vi "test_GetItemInformationFromProjects_SampleProject.vi"() -> (3 "Pass?":bool)   [LabVIEW 2019, in "Tests.SolutionBuilder.lvlib"]
uses:
  Tests.SolutionBuilder.lvlib
  SolutionBuilder/SolutionBuilder.lvclass
  SolutionBuilder/ProjectItem/ProjectItem.lvclass
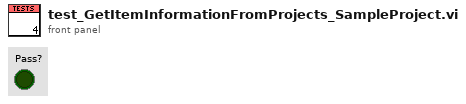
[diagram p1: front panel]
types:
  T1 = typedef "SolutionBuilder.lvlib/SolutionBuilder.lvclass/ProjectItemMap.ctl" = map{path, refnum<class "ProjectItem.lvclass">[]}
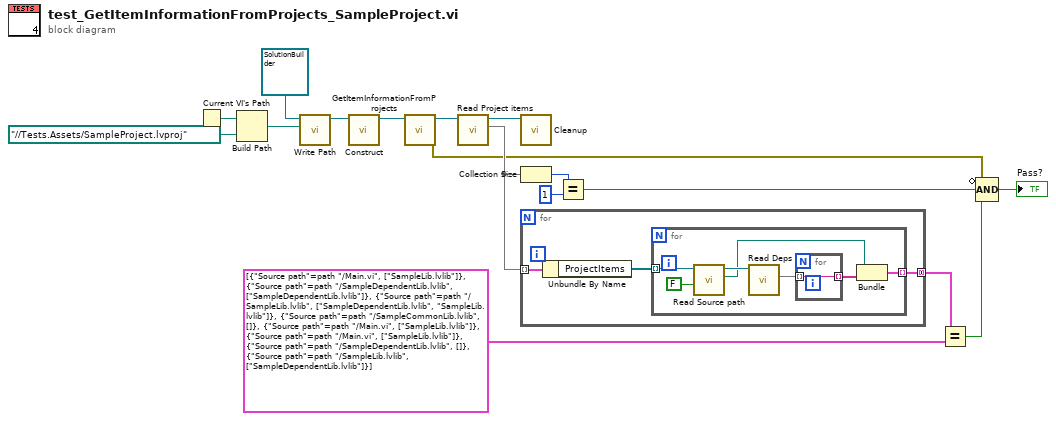
[diagram p0: block diagram]
diagram:
  n1 = Current VI's Path() -> (path=w16:path)
  n2 = Build Path(base path=w16, name or relative path=path "../../Tests.Assets/SampleProject.lvproj" ("Path")) -> (appended path=w14:path)
  n3 = call "Write Path.vi"("Path"=w14, "SolutionBuilder in"=refnum<class "SolutionBuilder.lvclass"> refnum) -> ("SolutionBuilder out"=w9:refnum<class "SolutionBuilder.lvclass">)  [unwired: 9 in]
  n4 = call "Construct.vi"("SolutionBuilder in"=w9) -> ("SolutionBuilder out"=w5:refnum<class "SolutionBuilder.lvclass">)  [unwired: 9 in, 1 out]
  n5 = call "GetItemInformationFromProjects.vi"("SolutionBuilder in"=w5) -> ("error out"=w2:errorcluster, "SolutionBuilder out"=w4:refnum<class "SolutionBuilder.lvclass">)  [unwired: 9 in]
  n6 = call "Read Project items.vi"("SolutionBuilder in"=w4) -> ("Project items"=w11:T1, "SolutionBuilder out"=w7:refnum<class "SolutionBuilder.lvclass">)  [unwired: 9 in]
  n7 = call "Cleanup.vi"("SolutionBuilder in"=w7) -> ()  [unwired: 9 in, 2 out]
  n8 = Collection Size(1:w11) -> (0:w13:i32)
  n9 = for {
    tunnel: w11 -> [w20] mode=indexing
    tunnel: [w18] -> w6 mode=concatenating
    n10 = Unbundle By Name(w20) -> ("ProjectItems"=w19:refnum<class "ProjectItem.lvclass">[])
    n11 = for {
      tunnel: w19 -> [w24] mode=indexing
      tunnel: [w25] -> w18 mode=indexing
      n12 = call "Read Source path.vi"("Force abs path? (T)"=FALSE, "ProjectItem in"=w24) -> ("Source path"=w22:path, "ProjectItem out"=w23:refnum<class "ProjectItem.lvclass">)  [unwired: 8 in]
      n13 = call "Read Deps.vi"("ProjectItem in"=w23) -> ("Deps"=w27:set{string})  [unwired: 9 in, 1 out]
      n14 = for {
        tunnel: w27 -> [w28] mode=indexing
        tunnel: [w28] -> w26 mode=indexing
      }
      n15 = Bundle("Source path"=w22, w26) -> (w25:cluster{"Source path":path, string[]})  [unwired: 1 in]
    }
  }
  n16 = Equal?(x=w13, y=1) -> (x = y?=w10:bool)
  n17 = Equal?(x=w6, y=cluster{"Source path":path, string[]}[] [{"Source path"=path "../Main.vi", ["SampleLib.lvlib"]}, {"Source path"=path "../SampleDependentLib.lvlib", ["SampleDependentLib.lvlib"]}, {"Source path"=path "../SampleLib.lvlib", ["SampleDependentLib.lvlib", "SampleLib.lvlib"]}, {"Source path"=path "../SampleCommonLib.lvlib", []}, {"Source path"=path "../Main.vi", ["SampleLib.lvlib"]}, {"Source path"=path "../Main.vi", ["SampleLib.lvlib"]}, {"Source path"=path "../SampleDependentLib.lvlib", []}, {"Source path"=path "../SampleLib.lvlib", ["SampleDependentLib.lvlib"]}] ("Array")) -> (x = y?=w8:bool)
  n18 = Compound Arithmetic op=AND(invert w2, w10, w8) -> (→"Pass?":bool)
